vi "tabla de índices de refracción.vi"() -> ()   [LabVIEW 2013]
panel:
  out "x*y":cdb
  out "numero":cdb
  out "String":string
  in  "Stop Button":bool
  in  "Índices de refracción":string[][](table)
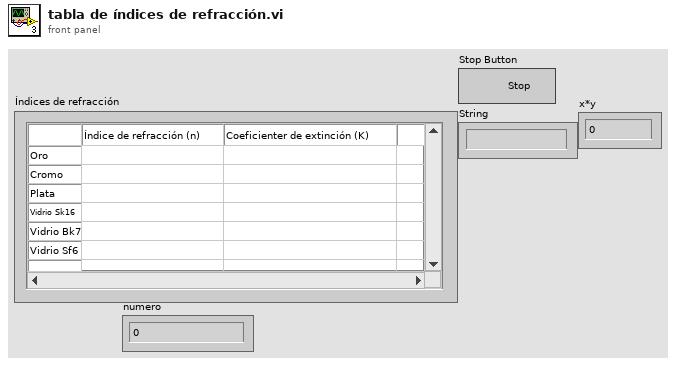
[diagram p1: front panel]
types:
  T1 = typedef "LVRowAndColumnTypeDef.ctl" = cluster{"Row":i32, "Column":i32}
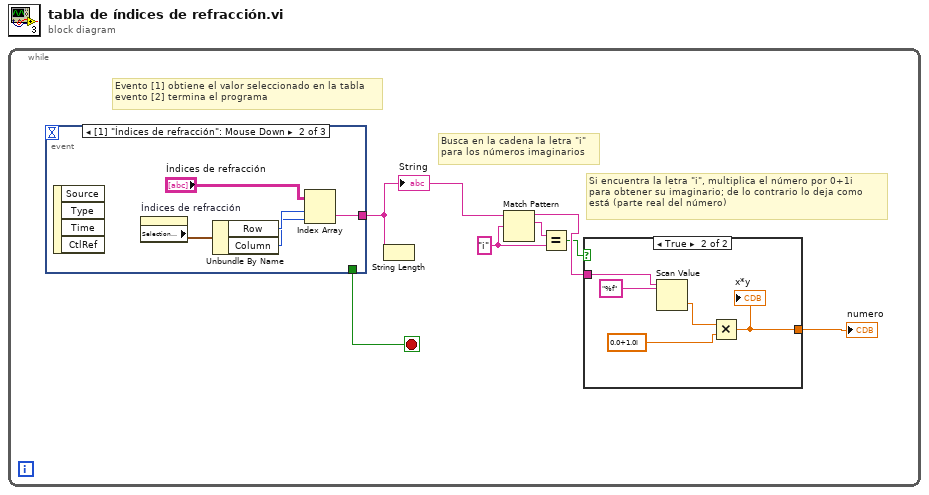
[diagram p0: block diagram]
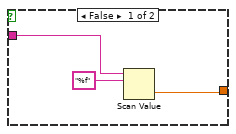
[diagram p2: hidden frame]
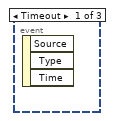
[diagram p3: hidden frame]
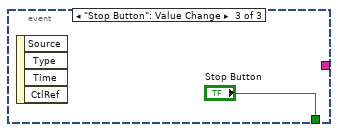
[diagram p4: hidden frame]
diagram:
  n1 = while {
    stop <- w7 stop-if-true
    w2 = "i" ("regular expression")
    # "Evento [1] obtiene el valor seleccionado en la tabla\nevento [2] termina el programa"
    # "Si encuentra la letra \"i\", multiplica el número por 0+1i \npara obtener su imaginario; de lo contrario lo deja como\nestá (parte real del número)"
    # "Busca en la cadena la letra \"i\" \npara los números imaginarios"
    n2 = event shown="[1] \"Índices de refracción\": Mouse Down" {
      selector: _ -> [_ _ _]
      dyn-events: _ -> [_ _ _]
      timeout: _ -> [_ _ _]
      tunnel: [_ w16 _] -> w4
      tunnel: [_ _ "Stop Button"] -> w7
      event Timeout {
        n3 = event-data() -> ()  [unwired: 1 in, 3 out]
      }
      event "Índices de refracción": Mouse Down {
        n4 = event-data() -> ()  [unwired: 1 in, 4 out]
        n5 = property on="Índices de refracción" class="Tbl (strict)"() -> ("Selection Start"=w20:T1)  [unwired: 2 in, 2 out]
        n6 = Unbundle By Name(w20) -> ("Row"=w18:i32, "Column"=w17:i32)
        n7 = Index Array(array="Índices de refracción", index (row)=w18, index (col)=w17) -> (element=w16:string)
      }
      event "Stop Button": Value Change {
        n8 = event-data() -> ()  [unwired: 1 in, 4 out]
      }
    }
    "String" <- w4
    n9 = String Length(string=w4) -> ()  [unwired: 1 out]
    n10 = Match Pattern(string=w4, regular expression=w2) -> (before substring=w5:string, match substring=w3:string)  [unwired: 1 in, 2 out]
    n11 = Equal?(x=w3, y=w2) -> (x = y?=w1:bool)
    n12 = case shown="True" w1 {
      tunnel: [w9 w12] -> w6
      tunnel: w5 -> [w8 w11]
      frame False {
        n13 = Scan Value(string=w8, format string="%f") -> (value=w9:dbl)  [unwired: 1 in, 1 out]
      }
      frame True {
        n14 = Scan Value(string=w11, format string="%f") -> (value=w13:dbl)  [unwired: 1 in, 1 out]
        n15 = Multiply(x=w13, y=csg 0.0+1.0i) -> (x*y=w12:cdb)
        "x*y" <- w12
      }
    }
    "numero" <- w6
  }
